vi "Create Plugins.vi"(5 "framework options":T1={"FIFO Options"={"Infinite Timeouts"=FALSE}, "Thread Options"={"Show FP On Call"=FALSE, "Close FP After Call"=FALSE, "Allow Debugging"=FALSE}, "Plugin Options"={"Default Components"=FALSE}, "Performance Options"={"Measure Period"=FALSE, "Measure Rx/Tx Duration"=FALSE}, "Data Server Options"={"Enable Data Server"=FALSE, "Period"=50}} {"Data Server Options"."Period" format="%d ms"}, 7 "Framework Configuration":refnum<class "Framework Configuration.lvclass">, 8 "error in (no error)":errorcluster, 10 "components directory":path, 11 "Framework in":refnum<class "Framework.lvclass">) -> (0 "error out":errorcluster, 1 "Plugin Threads":refnum<class "Plugin Thread.lvclass">[](array[class]), 2 "Plugins":refnum<class "Plugin.lvclass">[](array[class]), 3 "Framework out":refnum<class "Framework.lvclass">)   [LabVIEW 2019, in "DSF Core.lvlib" / "Framework.lvclass"]
uses:
  Framework.lvclass
  Plugin/Plugin.lvclass
  Configuration/Core/Framework/Framework Configuration.lvclass
  Thread/Plugin/Plugin Thread.lvclass
  Framework Options.ctl
  Typedefs/DSF FIFO Options.ctl
  Thread/Thread Options.ctl
  Typedefs/DSF Plugin Options.ctl
  Typedefs/DSF Performance Options.ctl
  Data Server Options.ctl
  Configuration/Core/Framework/Framework Configuration.lvclass/Framework Configuration.ctl
  Framework.lvclass/Framework.ctl
  Configuration/Core/Plugin/Plugin Configuration.lvclass/Plugin Configuration.ctl
  Component/Component.lvclass
  Configuration/Core/Plugin/Plugin Configuration.lvclass
  Component Loader/Component Loader.lvclass
  Transfer Group/Transfer Group.lvclass
  Thread/Thread.lvclass
  DSF Core.lvlib
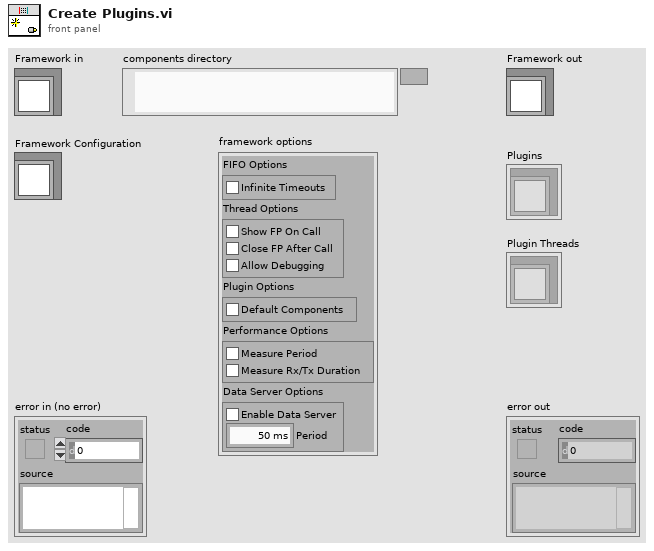
[diagram p1: front panel]
types:
  T1 = typedef "DSF Core.lvlib/Framework.lvclass/Framework Options.ctl" = cluster{"FIFO Options":T2, "Thread Options":T3, "Plugin Options":T4, "Performance Options":T5, "Data Server Options":T6}
  T2 = typedef "DSF Core.lvlib/Framework.lvclass/DSF FIFO Options.ctl" = cluster{"Infinite Timeouts":bool}
  T3 = typedef "DSF Core.lvlib/Thread.lvclass/Thread Options.ctl" = cluster{"Show FP On Call":bool, "Close FP After Call":bool, "Allow Debugging":bool}
  T4 = typedef "DSF Core.lvlib/Framework.lvclass/DSF Plugin Options.ctl" = cluster{"Default Components":bool}
  T5 = typedef "DSF Core.lvlib/DSF Performance Options.ctl" = cluster{"Measure Period":bool, "Measure Rx/Tx Duration":bool}
  T6 = typedef "DSF Core.lvlib/Framework.lvclass/Data Server Options.ctl" = cluster{"Enable Data Server":bool, "Period":u32}
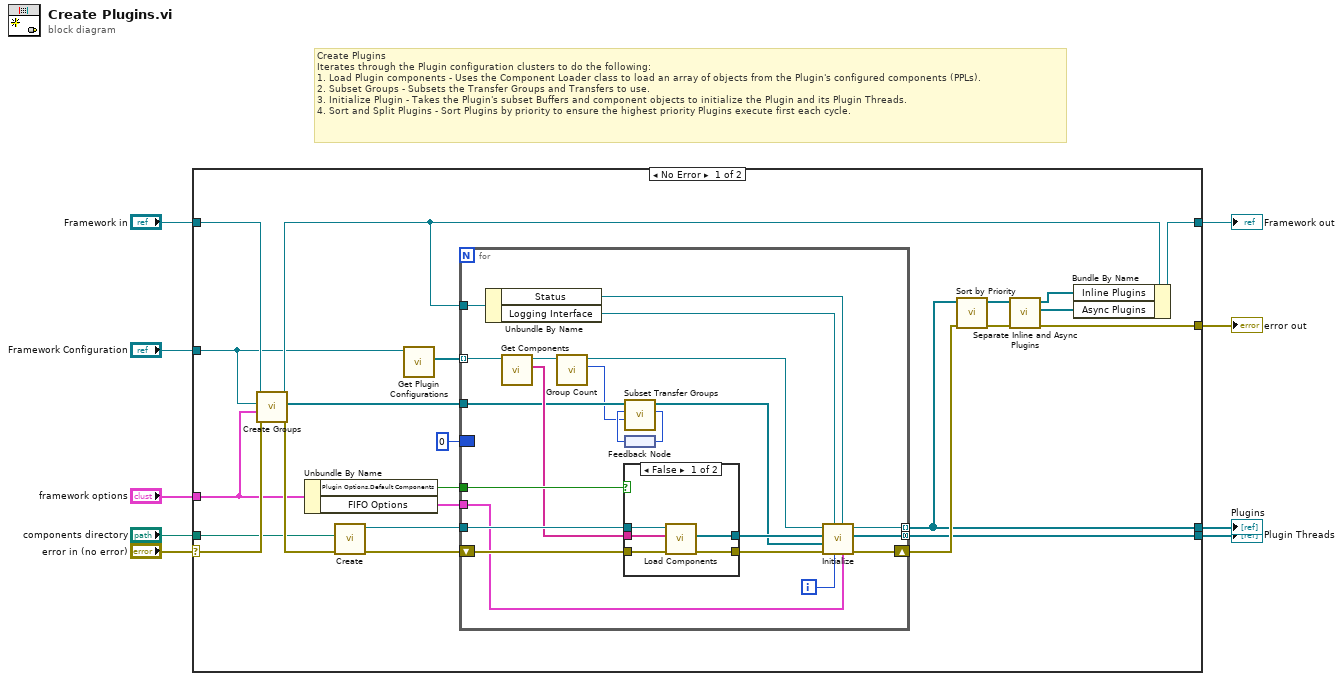
[diagram p0: block diagram]
diagram:
  # "Create Plugins\nIterates through the Plugin configuration clusters to do the following:\n1. Load Plugin components - Uses the Component Loader class to load an array of objects from the Plugin's configured components (PPLs).\n2. Subset Groups - Subsets the Transfer Groups and Transfers to use.\n3. Initialize Plugin - Takes the Plugin's subset Buffers and component objects to initialize the Plugin and its Plugin Threads.\n4. Sort and Split Plugins - Sort Plugins by priority to ensure the highest priority Plugins execute first each cycle."
  n1 = case shown="No Error" "error in (no error)" {
    selector: "error in (no error)" -> [w18 w61]
    tunnel: [w30 w61] -> w9
    tunnel: "Framework Configuration" -> [w16 _]
    tunnel: [w29 _] -> w7
    tunnel: [w22 _] -> w6
    tunnel: [w25 w62] -> w5
    tunnel: "framework options" -> [w10 _]
    tunnel: "Framework in" -> [w20 w62]
    tunnel: "components directory" -> [w11 _]
    frame No Error {
      n2 = call "Create Groups.vi"("error in (no error)"=w18, "framework options"=w10, "Framework Configuration"=w16, "Framework in"=w20) -> ("error out"=w17:errorcluster, "Transfer Groups"=w15:refnum<class "Transfer Group.lvclass">[], "Framework out"=w19:refnum<class "Framework.lvclass">)  [unwired: 5 in]
      n3 = Unbundle By Name(w10) -> ("Plugin Options.Default Components"=w13:bool, "FIFO Options"=w12:T2)
      n4 = call "Create.vi"("error in (no error)"=w17, "components directory"=w11) -> ("error out"=w32:errorcluster, "Component Loader out"=w23:refnum<class "Component Loader.lvclass">)  [unwired: 8 in]
      n5 = call "Get Plugin Configurations.vi"("Framework Configuration in"=w16) -> ("Plugin Configurations"=w21:refnum<class "Plugin Configuration.lvclass">[])  [unwired: 8 in, 2 out]
      n6 = for {
        shift-right: [w54] -> w31
        shift-left: w32 -> [w44]
        tunnel: w21 -> [w47] mode=indexing
        tunnel: w23 -> [w49]
        tunnel: [w53] -> w22 mode=indexing
        tunnel: [w52] -> w29 mode=concatenating
        tunnel: w19 -> [w50]
        tunnel: w15 -> [w37]
        border: 0 ("index") -> [_]
        tunnel: w13 -> [w42]
        tunnel: w12 -> [w41]
        i -> [w43]
        n7 = Unbundle By Name(w50) -> ("Status"=w39:refnum<class "Framework Status.lvclass">, "Logging Interface"=w45:refnum<class "Logging Interface.lvclass">)
        n8 = call "Get Components.vi"("Plugin Configuration in"=w47) -> ("components"=w40:string[], "Plugin Configuration out"=w46:refnum<class "Plugin Configuration.lvclass">)  [unwired: 8 in, 1 out]
        n9 = call-dynamic "Group Count.vi"("Plugin Configuration in"=w46) -> ("group count"=w34:i32, "Plugin Configuration out"=w38:refnum<class "Plugin Configuration.lvclass">)  [unwired: 8 in, 1 out]
        n10 = case shown="False" w42 {
          tunnel: [w59 w60] -> w48
          tunnel: w49 -> [w58 _]
          tunnel: w44 -> [w57 w60]
          tunnel: w40 -> [w56 _]
          tunnel: [w55 _] -> w51
          frame False {
            n11 = call "Load Components.vi"("error in (no error)"=w57, "component names"=w56, "Component Loader in"=w58) -> ("error out"=w59:errorcluster, "Components"=w55:refnum<class "Component.lvclass">[])  [unwired: 6 in, 1 out]
          }
          frame True {
            # "Skip loading components."
          }
        }
        n12 = feedback #1() -> (w35:i32)
        n13 = call "Subset Transfer Groups.vi"("count"=w34, "index"=w35, "Transfer Groups"=w37) -> ("index + count"=w33:i32, "subset Transfer Groups"=w36:refnum<class "Transfer Group.lvclass">[])  [unwired: 6 in, 1 out]
        n14 = feedback-in #1(w33) -> ()
        n15 = call "Initialize.vi"("FIFO Options"=w41, "Status"=w39, "id"=w43, "Logging Interface"=w45, "error in (no error)"=w48, "Transfer Groups"=w36, "Components"=w51, "Plugin Configuration"=w38) -> ("error out"=w54:errorcluster, "Plugin Threads"=w52:refnum<class "Plugin Thread.lvclass">[], "Plugin out"=w53:refnum<class "Plugin.lvclass">)  [unwired: 1 in]
      }
      n16 = call "Sort by Priority.vi"("error in (no error)"=w31, "Plugins in"=w22) -> ("error out"=w28:errorcluster, "Plugins out"=w24:refnum<class "Plugin.lvclass">[])  [unwired: 8 in]
      n17 = call "Separate Inline and Async Plugins.vi"("error in (no error)"=w28, "Plugins"=w24) -> ("error out"=w30:errorcluster, "Async Plugins"=w26:refnum<class "Plugin.lvclass">[], "Inline Plugins"=w27:refnum<class "Plugin.lvclass">[])  [unwired: 7 in]
      n18 = Bundle By Name(cluster=w19, "Inline Plugins"=w27, "Async Plugins"=w26) -> (w25:refnum<class "Framework.lvclass">)
    }
    frame Error {
    }
  }
  "error out" <- w9
  "Framework out" <- w5
  "Plugins" <- w6
  "Plugin Threads" <- w7
